vi "Parse Referential Element Data.vi"(7 "Tree In":refnum<class "Tree.lvclass">, 8 "error in":errorcluster, 11 "Element In":refnum<class "Tree.lvclass">) -> (0 "error out":errorcluster, 2 "Geometric":refnum<class "Geometric.lvclass">[](array[class]), 3 "Element Out":refnum<class "Tree.lvclass">, 5 "Tree Out":refnum<class "Tree.lvclass">)   [LabVIEW 2019, in "ParseGDSII.lvclass"]
uses:
  ParseGDSII.lvclass
  Tree/Tree.lvclass
  Elements/Geometric.lvclass
  Elements/Referential.lvclass
  DataTypes/Base/GDSII.DataType.lvclass
panel:
  out "Referential out":refnum<class "Referential.lvclass">
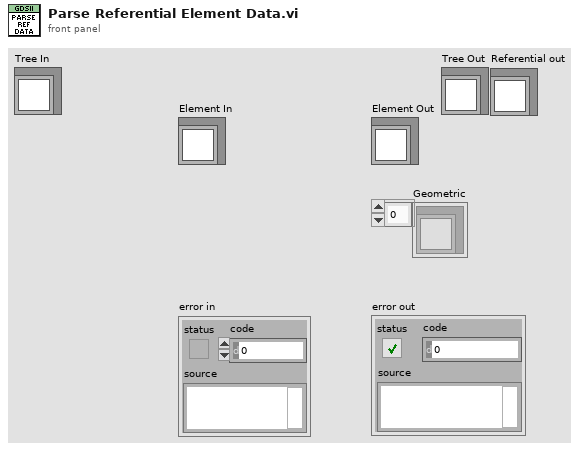
[diagram p1: front panel]
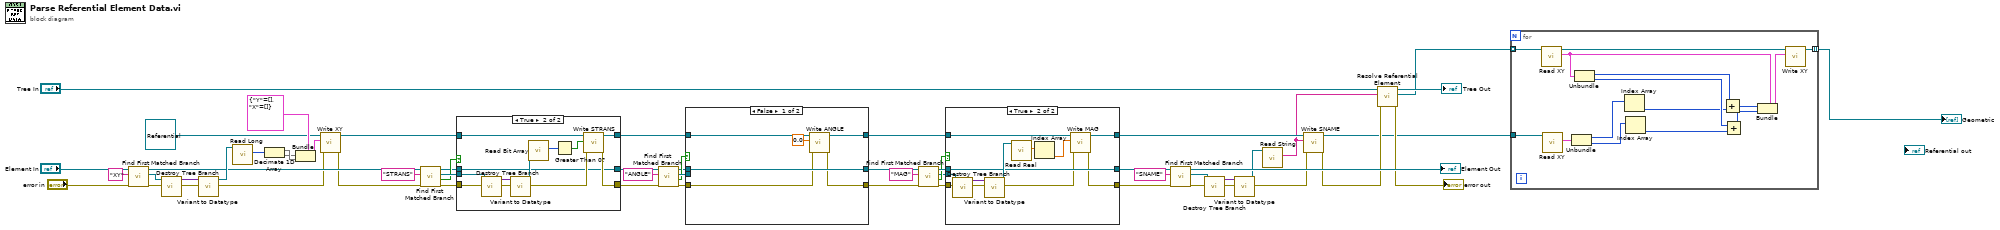
[diagram p0: block diagram]
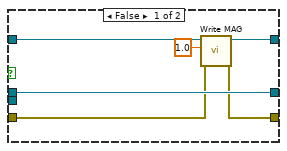
[diagram p3: hidden frame]
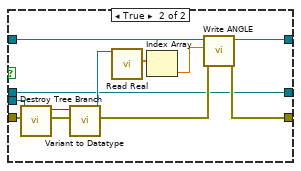
[diagram p4: hidden frame]
diagram:
  n1 = call "Find First Matched Branch.vi"("error in"="error in", "Branch Name Exact"="XY", "Tree in"="Element In") -> ("error out"=w42:errorcluster, "Matched Branch"=w57:refnum<class "Tree.lvclass">, "Tree out"=w53:refnum<class "Tree.lvclass">)  [unwired: 5 in, 1 out]
  n2 = call "Destroy Tree Branch.vi"("error in"=w42, "Tree in"=w57) -> ("error out"=w48:errorcluster, "Root"=w56:variant)  [unwired: 8 in]
  n3 = call "Variant to Datatype.vi"("error in"=w48, "Variant"=w56) -> ("error out"=w41:errorcluster, "DataType"=w55:refnum<class "GDSII.DataType.lvclass">)  [unwired: 8 in]
  n4 = call-dynamic "Read Long.vi"("GDSII.DataType in"=w55) -> ("Long"=w54:i32[])  [unwired: 9 in, 1 out]
  n5 = Decimate 1D Array(w54) -> (w45:i32[], w44:i32[])
  n6 = Bundle(cluster=cluster{"Y":i32[], "X":i32[]} {"Y"=[], "X"=[]} ("XY"), "Y"=w44, "X"=w45) -> (w43:cluster{"Y":i32[], "X":i32[]})
  n7 = call-dynamic "Write XY.vi"("error in (no error)"=w41, "XY"=w43, "Element in"=refnum<class "Referential.lvclass"> refnum ("Referential.lvclass")) -> ("error out"=w40:errorcluster, "Element out"=w34:refnum<class "Referential.lvclass">)  [unwired: 7 in]
  n8 = call "Find First Matched Branch.vi"("error in"=w40, "Branch Name Exact"="STRANS", "Tree in"=w53) -> ("error out"=w39:errorcluster, "Found?"=w3:bool, "Matched Branch"=w51:refnum<class "Tree.lvclass">, "Tree out"=w1:refnum<class "Tree.lvclass">)  [unwired: 5 in]
  n9 = case shown="True" w3 {
    tunnel: w51 -> [_ w72]
    tunnel: w39 -> [w60 w70]
    tunnel: [w60 w68] -> w35
    tunnel: w34 -> [w61 w67]
    tunnel: [w61 w63] -> w33
    tunnel: [w59 w62] -> w2
    tunnel: w1 -> [w59 w62]
    frame False {
    }
    frame True {
      n10 = call "Destroy Tree Branch.vi"("error in"=w70, "Tree in"=w72) -> ("error out"=w71:errorcluster, "Root"=w73:variant)  [unwired: 8 in]
      n11 = call "Variant to Datatype.vi"("error in"=w71, "Variant"=w73) -> ("error out"=w69:errorcluster, "DataType"=w66:refnum<class "GDSII.DataType.lvclass">)  [unwired: 8 in]
      n12 = call-dynamic "Read Bit Array.vi"("GDSII.DataType in"=w66) -> ("Bit Array"=w65:i16[])  [unwired: 9 in, 1 out]
      n13 = Greater Than 0?(x=w65) -> (x > 0?=w64:bool[])
      n14 = call-dynamic "Write STRANS.vi"("error in (no error)"=w69, "STRANS"=w64, "Referential in"=w67) -> ("error out"=w68:errorcluster, "Referential out"=w63:refnum<class "Referential.lvclass">)  [unwired: 7 in]
    }
  }
  n15 = call "Find First Matched Branch.vi"("error in"=w35, "Branch Name Exact"="ANGLE", "Tree in"=w2) -> ("error out"=w38:errorcluster, "Found?"=w32:bool, "Matched Branch"=w49:refnum<class "Tree.lvclass">, "Tree out"=w31:refnum<class "Tree.lvclass">)  [unwired: 5 in]
  n16 = case shown="False" w32 {
    tunnel: w49 -> [_ w90]
    tunnel: w38 -> [w76 w89]
    tunnel: [w77 w86] -> w23
    tunnel: w33 -> [w78 w82]
    tunnel: [w79 w81] -> w24
    tunnel: w31 -> [w79 w81]
    tunnel: [w74 w80] -> w25
    frame False {
      n17 = call-dynamic "Write ANGLE.vi"("error in (no error)"=w76, "ANGLE"=0.0, "Referential in"=w78) -> ("error out"=w77:errorcluster, "Referential out"=w74:refnum<class "Referential.lvclass">)  [unwired: 7 in]
    }
    frame True {
      n18 = call "Destroy Tree Branch.vi"("error in"=w89, "Tree in"=w90) -> ("error out"=w88:errorcluster, "Root"=w91:variant)  [unwired: 8 in]
      n19 = call "Variant to Datatype.vi"("error in"=w88, "Variant"=w91) -> ("error out"=w87:errorcluster, "DataType"=w85:refnum<class "GDSII.DataType.lvclass">)  [unwired: 8 in]
      n20 = call-dynamic "Read Real.vi"("GDSII.DataType in"=w85) -> ("Real"=w84:dbl[])  [unwired: 9 in, 1 out]
      n21 = Index Array(array=w84) -> (element=w83:dbl)  [unwired: 1 in]
      n22 = call-dynamic "Write ANGLE.vi"("error in (no error)"=w87, "ANGLE"=w83, "Referential in"=w82) -> ("error out"=w86:errorcluster, "Referential out"=w80:refnum<class "Referential.lvclass">)  [unwired: 7 in]
    }
  }
  n23 = call "Find First Matched Branch.vi"("error in"=w23, "Branch Name Exact"="MAG", "Tree in"=w24) -> ("error out"=w28:errorcluster, "Found?"=w29:bool, "Matched Branch"=w27:refnum<class "Tree.lvclass">, "Tree out"=w30:refnum<class "Tree.lvclass">)  [unwired: 5 in]
  n24 = case shown="True" w29 {
    tunnel: w27 -> [_ w108]
    tunnel: w28 -> [w96 w107]
    tunnel: [w95 w101] -> w12
    tunnel: [w97 w103] -> w16
    tunnel: w30 -> [w97 w103]
    tunnel: w25 -> [w94 w100]
    tunnel: [w93 w98] -> w22
    frame False {
      n25 = call-dynamic "Write MAG.vi"("error in (no error)"=w96, "MAG"=1.0 ("ANGLE"), "Referential in"=w94) -> ("error out"=w95:errorcluster, "Referential out"=w93:refnum<class "Referential.lvclass">)  [unwired: 7 in]
    }
    frame True {
      n26 = call "Destroy Tree Branch.vi"("error in"=w107, "Tree in"=w108) -> ("error out"=w106:errorcluster, "Root"=w109:variant)  [unwired: 8 in]
      n27 = call "Variant to Datatype.vi"("error in"=w106, "Variant"=w109) -> ("error out"=w102:errorcluster, "DataType"=w105:refnum<class "GDSII.DataType.lvclass">)  [unwired: 8 in]
      n28 = call-dynamic "Read Real.vi"("GDSII.DataType in"=w105) -> ("Real"=w104:dbl[])  [unwired: 9 in, 1 out]
      n29 = Index Array(array=w104) -> (element=w99:dbl)  [unwired: 1 in]
      n30 = call-dynamic "Write MAG.vi"("error in (no error)"=w102, "MAG"=w99, "Referential in"=w100) -> ("error out"=w101:errorcluster, "Referential out"=w98:refnum<class "Referential.lvclass">)  [unwired: 7 in]
    }
  }
  n31 = call "Find First Matched Branch.vi"("error in"=w12, "Branch Name Exact"="SNAME", "Tree in"=w16) -> ("error out"=w21:errorcluster, "Matched Branch"=w19:refnum<class "Tree.lvclass">, "Tree out"=→"Element Out":refnum<class "Tree.lvclass">)  [unwired: 5 in, 1 out]
  n32 = call "Destroy Tree Branch.vi"("error in"=w21, "Tree in"=w19) -> ("error out"=w20:errorcluster, "Root"=w18:variant)  [unwired: 8 in]
  n33 = call "Variant to Datatype.vi"("error in"=w20, "Variant"=w18) -> ("error out"=w14:errorcluster, "DataType"=w13:refnum<class "GDSII.DataType.lvclass">)  [unwired: 8 in]
  n34 = call-dynamic "Read String.vi"("GDSII.DataType in"=w13) -> ("String"=w9:string)  [unwired: 9 in, 1 out]
  n35 = call-dynamic "Write SNAME.vi"("error in (no error)"=w14, "SNAME"=w9, "Referential in"=w22) -> ("error out"=w8:errorcluster, "Referential out"=w5:refnum<class "Referential.lvclass">)  [unwired: 7 in]
  n36 = call "Resolve Referential Element.vi"("error in"=w8, "SNAME"=w9, "Tree In"="Tree In") -> ("error out"=→"error out":errorcluster, "Geometric"=w6:refnum<class "Geometric.lvclass">[], "Tree Out"=→"Tree Out":refnum<class "Tree.lvclass">)  [unwired: 6 in]
  n37 = for {
    tunnel: w6 -> [w123] mode=indexing
    tunnel: w5 -> [w124]
    tunnel: [w110] -> w4 mode=indexing
    n38 = call-dynamic "Read XY.vi"("Element in"=w123) -> ("XY"=w112:cluster{"Y":i32[], "X":i32[]}, "Element out"=w113:refnum<class "Geometric.lvclass">)  [unwired: 8 in, 1 out]
    n39 = call-dynamic "Read XY.vi"("Element in"=w124) -> ("XY"=w122:cluster{"Y":i32[], "X":i32[]})  [unwired: 8 in, 2 out]
    n40 = Unbundle(w122) -> ("Y"=w115:i32[], "X"=w117:i32[])
    n41 = Unbundle(w112) -> ("Y"=w121:i32[], "X"=w120:i32[])
    n42 = Index Array(array=w115) -> (element=w114:i32)  [unwired: 1 in]
    n43 = Index Array(array=w117) -> (element=w116:i32)  [unwired: 1 in]
    n44 = Add(x=w121, y=w114) -> (x+y=w119:i32[])
    n45 = Add(x=w120, y=w116) -> (x+y=w118:i32[])
    n46 = Bundle(cluster=w112, "Y"=w119, "X"=w118) -> (w111:cluster{"Y":i32[], "X":i32[]})
    n47 = call-dynamic "Write XY.vi"("XY"=w111, "Element in"=w113) -> ("Element out"=w110:refnum<class "Geometric.lvclass">)  [unwired: 8 in, 1 out]
  }
  "Geometric" <- w4
